vi "find_period.vi"(8 "error in (no error)":errorcluster, 9 "Amplitude Thresh":dbl format="%#_13g", 10 "Amplitude":dbl, 11 "VISA In":refnum<visa-resource-name>) -> (0 "error out":errorcluster, 1 "Time Low":dbl, 2 "Time High":dbl, 3 "VISA Out":refnum<visa-resource-name>, 4 "Pulse Status":bool, 5 "Time Out":dbl)   [LabVIEW 2011]
panel:
  in  "Query String":string
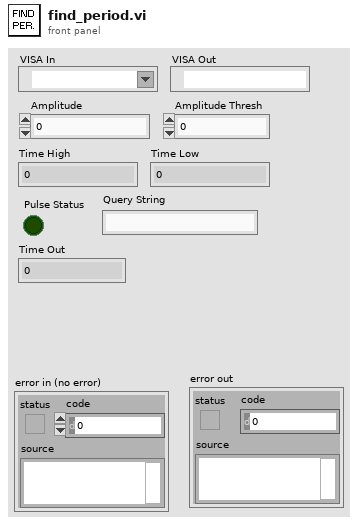
[diagram p1: front panel]
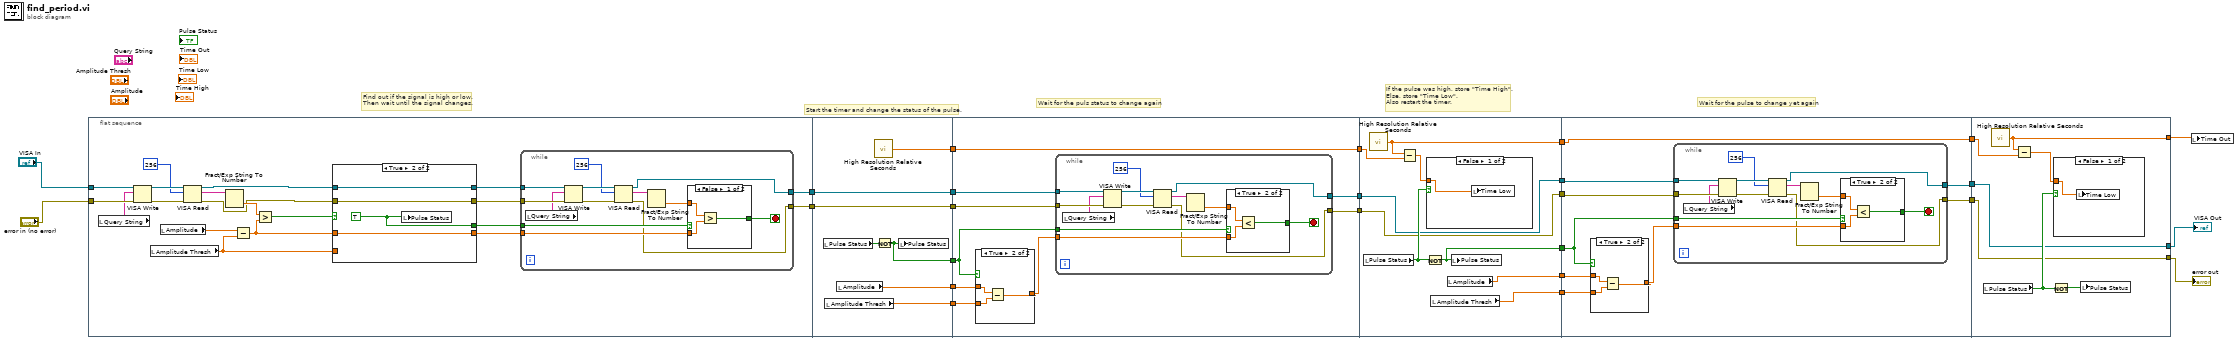
[diagram p0: block diagram]
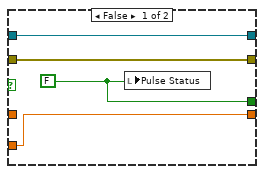
[diagram p2: hidden frame]
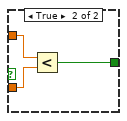
[diagram p3: hidden frame]
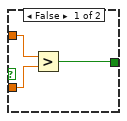
[diagram p5: hidden frame]
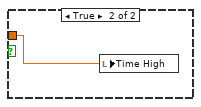
[diagram p6: hidden frame]
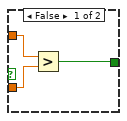
[diagram p8: hidden frame]
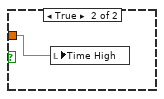
[diagram p9: hidden frame]
diagram:
  # "Wait for the pulse to change yet again"
  # "If the pulse was high, store \"Time High\".\nElse, store \"Time Low\".\nAlso restart the timer."
  # "Wait for the puls status to change again"
  # "Start the timer and change the status of the pulse."
  # "Find out if the signal is high or low.\nThen wait until the signal changes."
  n1 = flat-sequence {
    tunnel: "VISA In" -> [w30]
    tunnel: "error in (no error)" -> [w29]
    tunnel: [w28] -> w23
    tunnel: [w27] -> w22
    tunnel: w23 -> [w78]
    tunnel: w22 -> [w77]
    tunnel: [w73] -> w21
    tunnel: [w78] -> w20
    tunnel: [w77] -> w19
    tunnel: [w76] -> w18
    tunnel: [w75] -> w17
    tunnel: [w74] -> w16
    tunnel: w21 -> [w82]
    tunnel: w20 -> [w88]
    tunnel: w19 -> [w87]
    tunnel: w18 -> [w86]
    tunnel: w17 -> [w85]
    tunnel: w16 -> [w84]
    tunnel: [w82] -> w15
    tunnel: [w81] -> w14
    tunnel: [w80] -> w13
    tunnel: w15 -> [w120]
    tunnel: w14 -> [w117]
    tunnel: w13 -> [w116]
    tunnel: [w117] -> w12
    tunnel: [w116] -> w11
    tunnel: [w115] -> w10
    tunnel: [w114] -> w9
    tunnel: [w113] -> w8
    tunnel: [w112] -> w7
    tunnel: w12 -> [w130]
    tunnel: w11 -> [w129]
    tunnel: w10 -> [w123]
    tunnel: w9 -> [w128]
    tunnel: w8 -> [w127]
    tunnel: w7 -> [w126]
    tunnel: [w125] -> w6
    tunnel: [w124] -> w5
    tunnel: [w123] -> w4
    tunnel: w6 -> [w156]
    tunnel: w5 -> [w155]
    tunnel: w4 -> [w161]
    tunnel: [w157] -> w1
    tunnel: [w156] -> w2
    tunnel: [w155] -> w3
    frame #0 {
      n2 = local read "Query String"() -> (w26:string)
      n3 = VISA Write(VISA resource name=w30, write buffer=w26, error in (no error)=w29) -> (VISA resource name out=w45:refnum<visa-resource-name>, error out=w44:errorcluster)  [unwired: 1 out]
      n4 = local read "Amplitude Thresh"() -> (w37:dbl)
      n5 = local read "Amplitude"() -> (w41:dbl)
      n6 = VISA Read(VISA resource name=w45, byte count=u32 256, error in (no error)=w44) -> (VISA resource name out=w35:refnum<visa-resource-name>, read buffer=w42:string, error out=w34:errorcluster)  [unwired: 1 out]
      n7 = Fract/Exp String To Number(string=w42) -> (number=w40:dbl)  [unwired: 3 in, 1 out]
      n8 = Subtract(x=w41, y=w37) -> (x-y=w38:dbl)
      n9 = Greater?(x=w40, y=w38) -> (0:w39:bool)
      n10 = case shown="True" w39 {
        tunnel: [w49 w53] -> w36
        tunnel: w38 -> [_ w53]
        tunnel: w37 -> [w49 _]
        tunnel: w35 -> [w47 w52]
        tunnel: w34 -> [w48 w51]
        tunnel: [w48 w51] -> w32
        tunnel: [w47 w52] -> w33
        tunnel: [w46 w50] -> w31
        frame False {
          w46 = FALSE
          n11 = local write "Pulse Status"(w46) -> ()
        }
        frame True {
          w50 = TRUE
          n12 = local write "Pulse Status"(w50) -> ()
        }
      }
      n13 = while {
        tunnel: w36 -> [w59]
        tunnel: w33 -> [w62]
        tunnel: w32 -> [w61]
        tunnel: w31 -> [w60]
        tunnel: [w56] -> w28
        tunnel: [w55] -> w27
        stop <- w57 stop-if-true
        n14 = local read "Query String"() -> (w54:string)
        n15 = VISA Write(VISA resource name=w62, write buffer=w54, error in (no error)=w61) -> (VISA resource name out=w66:refnum<visa-resource-name>, error out=w65:errorcluster)  [unwired: 1 out]
        n16 = VISA Read(VISA resource name=w66, byte count=u32 256, error in (no error)=w65) -> (VISA resource name out=w56:refnum<visa-resource-name>, read buffer=w63:string, error out=w55:errorcluster)  [unwired: 1 out]
        n17 = Fract/Exp String To Number(string=w63) -> (number=w58:dbl)  [unwired: 3 in, 1 out]
        n18 = case shown="False" w60 {
          tunnel: w59 -> [w69 w71]
          tunnel: w58 -> [w68 w72]
          tunnel: [w67 w70] -> w57
          frame False {
            n19 = Greater?(x=w68, y=w69) -> (0:w67:bool)
          }
          frame True {
            n20 = Less?(x=w72, y=w71) -> (x < y?=w70:bool)
          }
        }
      }
    }
    frame #1 {
      n21 = local read "Pulse Status"() -> (w79:bool)
      n22 = local read "Amplitude Thresh"() -> (w74:dbl)
      n23 = local read "Amplitude"() -> (w75:dbl)
      n24 = call <vilib>:"High Resolution Relative Seconds.vi"() -> ("relative seconds"=w73:dbl)
      n25 = Not(x=w79) -> (.not. x?=w76:bool)
      n26 = local write "Pulse Status"(w76) -> ()
    }
    frame #2 {
      n27 = case shown="True" w86 {
        tunnel: w85 -> [_ w92]
        tunnel: w84 -> [w89 w91]
        tunnel: [w89 w90] -> w83
        frame False {
        }
        frame True {
          n28 = Subtract(x=w92, y=w91) -> (x-y=w90:dbl)
        }
      }
      n29 = while {
        tunnel: w83 -> [w98]
        tunnel: w88 -> [w101]
        tunnel: w87 -> [w100]
        tunnel: w86 -> [w99]
        tunnel: [w95] -> w81
        tunnel: [w94] -> w80
        stop <- w96 stop-if-true
        n30 = local read "Query String"() -> (w93:string)
        n31 = VISA Write(VISA resource name=w101, write buffer=w93, error in (no error)=w100) -> (VISA resource name out=w105:refnum<visa-resource-name>, error out=w104:errorcluster)  [unwired: 1 out]
        n32 = VISA Read(VISA resource name=w105, byte count=u32 256, error in (no error)=w104) -> (VISA resource name out=w95:refnum<visa-resource-name>, read buffer=w102:string, error out=w94:errorcluster)  [unwired: 1 out]
        n33 = Fract/Exp String To Number(string=w102) -> (number=w97:dbl)  [unwired: 3 in, 1 out]
        n34 = case shown="True" w99 {
          tunnel: w98 -> [w108 w110]
          tunnel: w97 -> [w107 w111]
          tunnel: [w106 w109] -> w96
          frame False {
            n35 = Greater?(x=w107, y=w108) -> (0:w106:bool)
          }
          frame True {
            n36 = Less?(x=w111, y=w110) -> (x < y?=w109:bool)
          }
        }
      }
    }
    frame #3 {
      n37 = local read "Pulse Status"() -> (w119:bool)
      n38 = call <vilib>:"High Resolution Relative Seconds.vi"() -> ("relative seconds"=w115:dbl)
      n39 = Subtract(x=w115, y=w120) -> (x-y=w118:dbl)
      n40 = case shown="False" w119 {
        tunnel: w118 -> [w121 w122]
        frame False {
          n41 = local write "Time Low"(w121) -> ()
        }
        frame True {
          n42 = local write "Time High"(w122) -> ()
        }
      }
      n43 = Not(x=w119) -> (.not. x?=w112:bool)
      n44 = local read "Amplitude Thresh"() -> (w113:dbl)
      n45 = local read "Amplitude"() -> (w114:dbl)
      n46 = local write "Pulse Status"(w112) -> ()
    }
    frame #4 {
      n47 = case shown="True" w126 {
        tunnel: w128 -> [_ w135]
        tunnel: w127 -> [w132 w134]
        tunnel: [w132 w133] -> w131
        frame False {
        }
        frame True {
          n48 = Subtract(x=w135, y=w134) -> (x-y=w133:dbl)
        }
      }
      n49 = while {
        tunnel: w131 -> [w141]
        tunnel: w130 -> [w144]
        tunnel: w129 -> [w143]
        tunnel: w126 -> [w142]
        tunnel: [w138] -> w125
        tunnel: [w137] -> w124
        stop <- w139 stop-if-true
        n50 = local read "Query String"() -> (w136:string)
        n51 = VISA Write(VISA resource name=w144, write buffer=w136, error in (no error)=w143) -> (VISA resource name out=w148:refnum<visa-resource-name>, error out=w147:errorcluster)  [unwired: 1 out]
        n52 = VISA Read(VISA resource name=w148, byte count=u32 256, error in (no error)=w147) -> (VISA resource name out=w138:refnum<visa-resource-name>, read buffer=w145:string, error out=w137:errorcluster)  [unwired: 1 out]
        n53 = Fract/Exp String To Number(string=w145) -> (number=w140:dbl)  [unwired: 3 in, 1 out]
        n54 = case shown="True" w142 {
          tunnel: w141 -> [w151 w153]
          tunnel: w140 -> [w150 w154]
          tunnel: [w149 w152] -> w139
          frame False {
            n55 = Greater?(x=w150, y=w151) -> (0:w149:bool)
          }
          frame True {
            n56 = Less?(x=w154, y=w153) -> (x < y?=w152:bool)
          }
        }
      }
    }
    frame #5 {
      n57 = local read "Pulse Status"() -> (w159:bool)
      n58 = call <vilib>:"High Resolution Relative Seconds.vi"() -> ("relative seconds"=w157:dbl)
      n59 = Subtract(x=w157, y=w161) -> (x-y=w158:dbl)
      n60 = Not(x=w159) -> (.not. x?=w160:bool)
      n61 = case shown="False" w159 {
        tunnel: w158 -> [w162 w163]
        frame False {
          n62 = local write "Time Low"(w162) -> ()
        }
        frame True {
          n63 = local write "Time High"(w163) -> ()
        }
      }
      n64 = local write "Pulse Status"(w160) -> ()
    }
  }
  n65 = local write "Time Out"(w1) -> ()
  "VISA Out" <- w2
  "error out" <- w3
